vi "Data Server.vi"(8 "error in (no error)":errorcluster, 11 "Node Ptr":T1 format="%.0x") -> (0 "error out":errorcluster)   [LabVIEW 2021, in "gRPC Data Server System Explorer.lvlib"]
uses:
  gRPC Data Server System Explorer.lvlib
  <vilib>/NI VeriStand/Custom Device API/Custom Device Item Ref.ctl
  <vilib>/Utility/file.llb/Read Delimited Spreadsheet (string).vi
  <vilib>/Utility/file.llb/Write Delimited Spreadsheet (string).vi
  <vilib>/NI VeriStand/Custom Device API/Custom Device API.lvlib
  Shared/gRPC Data Server Shared.lvlib
panel:
  in  "Data":string[][](table)
  in  "Import":bool
  in  "Export":bool
  in  "SHDocVw.IWebBrowser":refnum<k7>(container)
  in  "Specific Header":cluster{"Section Name":string}={"Section Name"="Data in Memory"}
  in  "General Header":cluster{"Section Name":string}={"Section Name"="General Page Settings"}
  in  "Description":string
  in  "Name":string
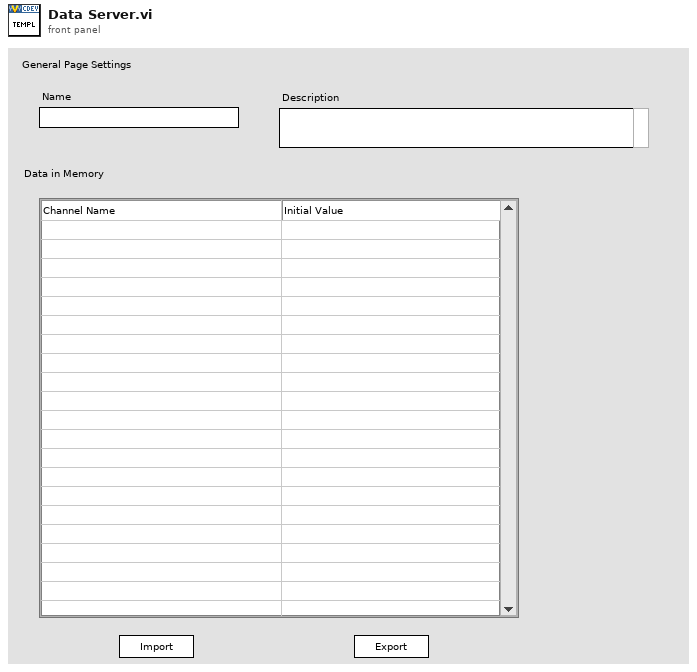
[diagram p1: front panel]
types:
  T1 = typedef "Custom Device API.lvlib/Custom Device Item Ref.ctl" = u64
  T2 = typedef "Custom Device API.lvlib/Custom Device Item Info.ctl" = cluster{"Name":string, "Is Channel":bool, "GUID":string, "Is Waveform":bool}
  T3 = typedef "gRPC Data Server Shared.lvlib/Compiled.Settings.ctl" = cluster{"Name":string, "Server Address":string, "Async?":bool, "Key File":path, "Cert File":path, "Channel Name":string[], "Initial Value":string[]}
  T4 = typedef "Custom Device API.lvlib/Custom Device Commands.ctl" = enum16{"Default", "Item renamed", "Shutdown", "Dynamic button pressed"}
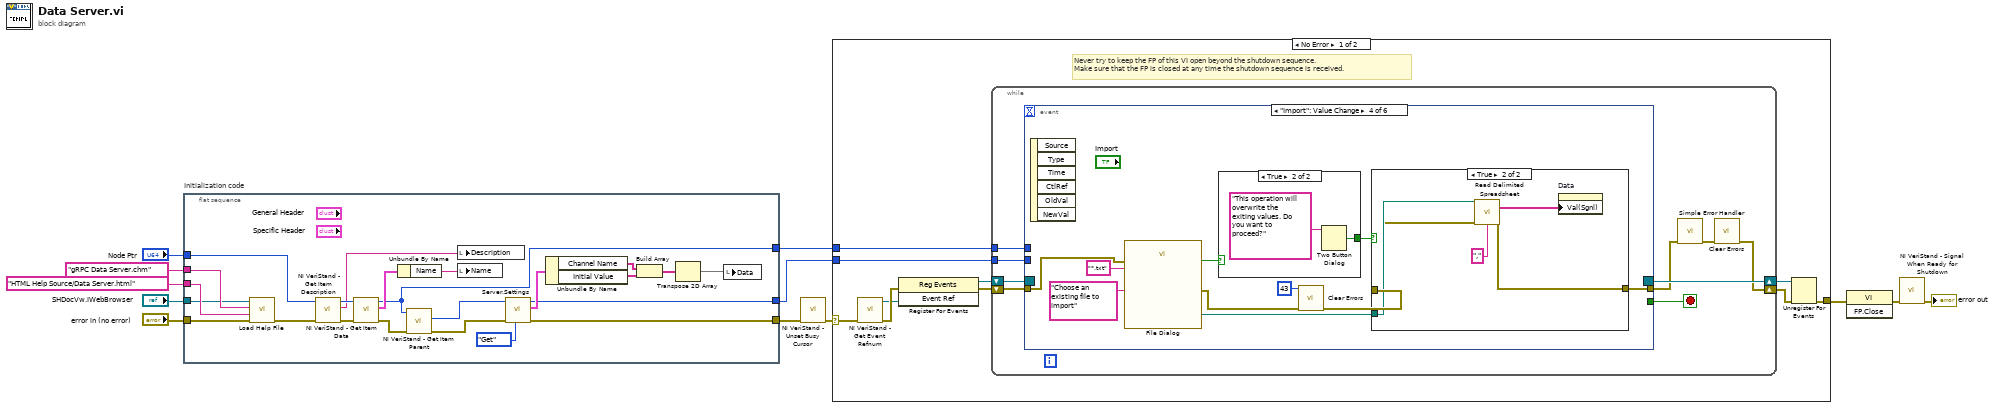
[diagram p0: block diagram]
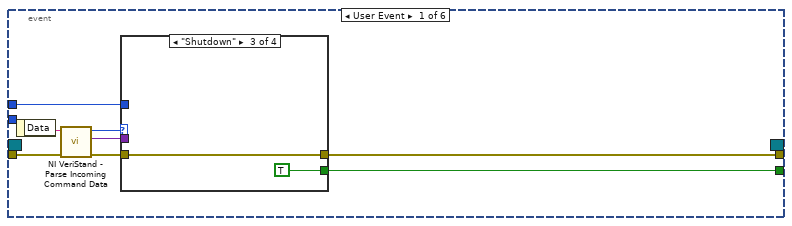
[diagram p2: hidden frame]
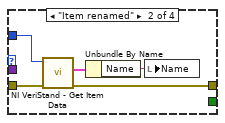
[diagram p4: hidden frame]
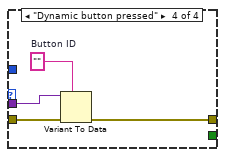
[diagram p5: hidden frame]
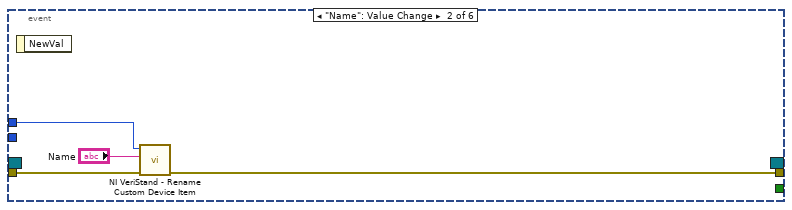
[diagram p6: hidden frame]
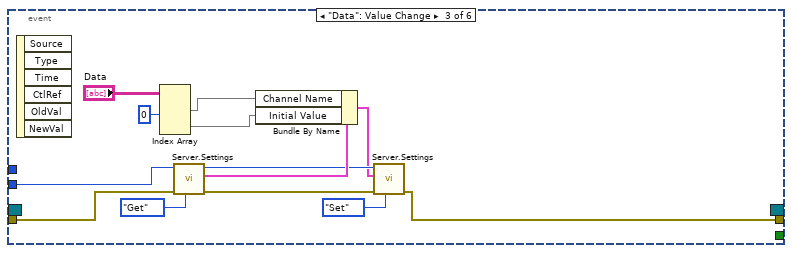
[diagram p7: hidden frame]
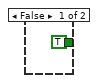
[diagram p9: hidden frame]
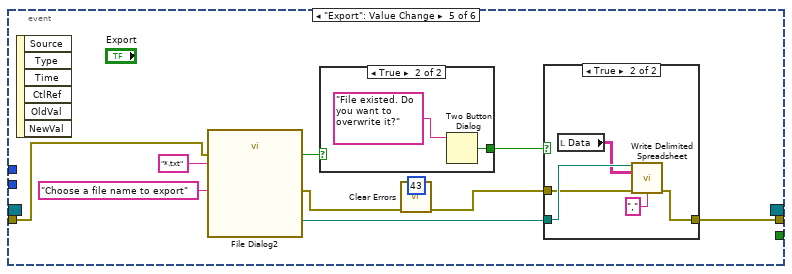
[diagram p10: hidden frame]
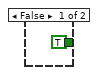
[diagram p12: hidden frame]
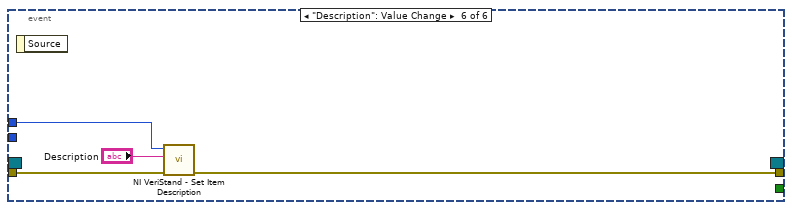
[diagram p13: hidden frame]
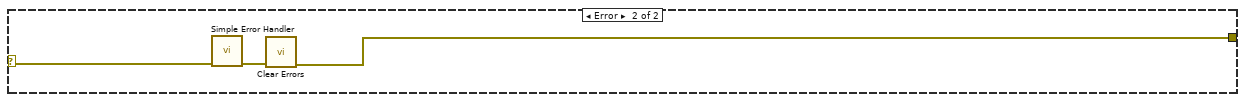
[diagram p14: hidden frame]
diagram:
  n1 = flat-sequence "Initialization code" {
    tunnel: "error in (no error)" -> [w29]
    tunnel: "Node Ptr" -> [w32]
    tunnel: [w23] -> w8
    tunnel: [w17] -> w5
    tunnel: "SHDocVw.IWebBrowser" -> [w25]
    tunnel: "HTML Help Source/Data Server.html" ("CD_CHM_Section") -> [w27]
    tunnel: "gRPC Data Server.chm" ("CD_CHM_FileName") -> [w26]
    tunnel: [w13] -> w1
    frame #0 {
      n2 = call "Load Help File.vi"("error in (no error)"=w29, "HTML File to Load"=w27, "Main CHM File"=w26, "Browser"=w25) -> ("error out"=w28:errorcluster)  [unwired: 7 in]
      n3 = call <vilib>:"NI VeriStand - Get Item Description.vi"("error in (no error)"=w28, "Item Ref in"=w32) -> ("error out"=w34:errorcluster, "Description"=w30:string, "Item Ref out"=w35:T1)  [unwired: 7 out]
      n4 = call <vilib>:"NI VeriStand - Get Item Data.vi"("error in (no error)"=w34, "Item Ref in"=w35) -> ("error out"=w16:errorcluster, "Item Info"=w33:T2, "Item Ref out"=w17:T1)  [unwired: 7 out]
      n5 = Unbundle By Name(w33) -> ("Name"=w31:string)
      n6 = call <vilib>:"NI VeriStand - Get Item Parent.vi"("error in (no error)"=w16, "Item Ref in"=w17) -> ("error out"=w14:errorcluster, "Parent Ref"=w15:T1)  [unwired: 6 in, 2 out]
      n7 = local write "Description"(w30) -> ()
      n8 = local write "Name"(w31) -> ()
      n9 = call "Server.Settings.vi"("Action"=enum8{"Get", "Set"}."Get", "error in (no error)"=w14, "Parent Ref in"=w15) -> ("error out"=w23:errorcluster, "Settings Out"=w22:T3, "Item Ref out"=w13:T1)  [unwired: 6 in]
      n10 = Unbundle By Name(w22) -> ("Channel Name"=w21:string[], "Initial Value"=w20:string[])
      n11 = Build Array(w21, w20) -> (w19:string[][])
      n12 = Transpose 2D Array(2D array=w19) -> (transposed array=w18:string[][])
      n13 = local write "Data"(w18) -> ()
    }
  }
  n14 = call <vilib>:"NI VeriStand - Unset Busy Cursor.vi"("error in (no error)"=w8) -> ("error out"=w7:errorcluster)  [unwired: 10 out]
  n15 = case shown="No Error" w7 {
    selector: w7 -> [w37 w136]
    tunnel: [w42 w134] -> w12
    tunnel: w5 -> [w38 _]
    tunnel: w1 -> [w36 _]
    frame No Error {
      # "Never try to keep the FP of this VI open beyond the shutdown sequence.\nMake sure that the FP is closed at any time the shutdown sequence is received."
      n16 = call <vilib>:"NI VeriStand - Get Event Refnum.vi"("error in (no error)"=w37) -> ("error out"=w45:errorcluster, "Event Ref"=w41:refnum<user-event>)  [unwired: 9 out]
      n17 = register-events(error in=w45, w41) -> (reference out=w39:refnum<event-registration>, error out=w40:errorcluster)  [unwired: 1 in]
      n18 = while {
        tunnel: w38 -> [w50]
        shift-right: [w47] -> w43
        shift-left: w40 -> [w53]
        shift-right: [w54] -> w44
        shift-left: w39 -> [w52]
        tunnel: w36 -> [w46]
        stop <- w51 stop-if-true
        n19 = event shown="[3] \"Import\": Value Change" {
          selector: w52 -> [_ _ _ _ _ _]
          dyn-events: [_ _ _ _ _ _] -> w54
          timeout: _ -> [_ _ _ _ _ _]
          tunnel: w53 -> [w62 w78 w85 w99 w115 w132]
          tunnel: [w58 _ _ _ _ _] -> w51
          tunnel: [w57 w77 w84 w95 w114 w131] -> w49
          tunnel: w50 -> [w56 w76 _ _ _ w133]
          tunnel: w46 -> [_ _ w79 _ _ _]
          event User Event {
            n20 = event-data() -> ("Data"=w61:string)  [unwired: 1 out]
            n21 = call <vilib>:"NI VeriStand - Parse Incoming Command Data.vi"("error in (no error)"=w62, "Incoming data"=w61) -> ("error out"=w60:errorcluster, "Outgoing data"=w55:variant, "Action"=w59:T4)  [unwired: 7 out]
            n22 = case shown="\"Shutdown\"" w59 {
              tunnel: w60 -> [w63 w68 w69 w74]
              tunnel: [_ _ TRUE _] -> w58
              tunnel: [w63 w65 w69 w71] -> w57
              tunnel: w56 -> [_ w67 _ _]
              tunnel: w55 -> [_ _ _ w73]
              frame "Default", Default {
              }
              frame "Item renamed" {
                n23 = call <vilib>:"NI VeriStand - Get Item Data.vi"("error in (no error)"=w68, "Item Ref in"=w67) -> ("error out"=w65:errorcluster, "Item Info"=w66:T2)  [unwired: 8 out]
                n24 = Unbundle By Name(w66) -> ("Name"=w64:string)
                n25 = local write "Name"(w64) -> ()
              }
              frame "Shutdown" {
              }
              frame "Dynamic button pressed" {
                w72 = ""  # Button ID
                n26 = Variant To Data(error in=w74, type=w72, Variant=w73) -> (error out=w71:errorcluster)  [unwired: 1 out]
              }
            }
          }
          event "Name": Value Change {
            n27 = event-data() -> ()  [unwired: 2 out]
            n28 = call <vilib>:"NI VeriStand - Rename Custom Device Item.vi"("error in (no error)"=w78, "New Name"="Name", "Item Ref in"=w76) -> ("error out"=w77:errorcluster)  [unwired: 1 in, 7 out]
          }
          event "Data": Value Change {
            n29 = event-data() -> ()  [unwired: 7 out]
            n30 = Index Array(array="Data", index (col) #1=0 ("disabled index (col)")) -> (element #1=w81:string[], element #2=w80:string[])  [unwired: 3 in]
            n31 = call "Server.Settings.vi"("Action"=enum8{"Get", "Set"}."Get", "error in (no error)"=w85, "Parent Ref in"=w79) -> ("error out"=w88:errorcluster, "Settings Out"=w90:T3, "Item Ref out"=w89:T1)  [unwired: 6 in]
            n32 = Bundle By Name(cluster=w90, "Channel Name"=w81, "Initial Value"=w80) -> (w87:T3)
            n33 = call "Server.Settings.vi"("Action"=enum8{"Get", "Set"}."Set", "error in (no error)"=w88, "Settings In"=w87, "Parent Ref in"=w89) -> ("error out"=w84:errorcluster)  [unwired: 5 in, 2 out]
          }
          event "Import": Value Change {
            n34 = event-data() -> ()  [unwired: 7 out]
            n35 = call "File Dialog"("prompt"="Choose an existing file to import", "error in"=w99, "pattern (all files)"="*.txt" ("default name")) -> ("selected path"=w96:path, "exists"=w97:bool, "error out"=w94:errorcluster)  [unwired: 9 in, 1 out]
            n36 = case shown="True" w97 {
              tunnel: [TRUE ("T button?") w109] -> w98
              frame False {
              }
              frame True {
                n37 = Two Button Dialog(message="This operation will overwrite the exiting values. Do you want to proceed?") -> (T button?=w109:bool)  [unwired: 2 in]
              }
            }
            n38 = call <vilib>:"Clear Errors.vi"("error in (no error)"=w94, "specific error code to clear (0: all)"=43) -> ("error out"=w93:errorcluster)  [unwired: 4 in, 1 out]
            n39 = case shown="True" w98 {
              tunnel: w96 -> [_ w107]
              tunnel: w93 -> [w102 w105]
              tunnel: [w102 w104] -> w95
              frame False {
              }
              frame True {
                n40 = call-poly <vilib>:"Read Delimited Spreadsheet.vi"("file path (dialog if empty)"=w107, "error in (no error)"=w105, "delimiter (\\t)"="," ("delimiter (\\t)")) -> ("all rows"=w103:string[][], "error out"=w104:errorcluster)  [unwired: 7 in, 4 out]
                n41 = property on="Data" class="Tbl (strict)"("Val(Sgnl)"=w103) -> ()  [unwired: 2 in, 2 out]
              }
            }
          }
          event "Export": Value Change {
            n42 = event-data() -> ()  [unwired: 7 out]
            n43 = call "File Dialog2"("prompt"="Choose a file name to export", "error in"=w115, "pattern (all files)"="*.txt" ("default name")) -> ("selected path"=w116:path, "exists"=w118:bool, "error out"=w112:errorcluster)  [unwired: 9 in, 1 out]
            n44 = case shown="True" w118 {
              tunnel: [TRUE ("T button?") w128] -> w117
              frame False {
              }
              frame True {
                n45 = Two Button Dialog(message="File existed. Do you want to overwrite it?") -> (T button?=w128:bool)  [unwired: 2 in]
              }
            }
            n46 = call <vilib>:"Clear Errors.vi"("error in (no error)"=w112, "specific error code to clear (0: all)"=43) -> ("error out"=w111:errorcluster)  [unwired: 4 in, 1 out]
            n47 = case shown="True" w117 {
              tunnel: w116 -> [_ w126]
              tunnel: w111 -> [w121 w123]
              tunnel: [w121 w122] -> w114
              frame False {
              }
              frame True {
                n48 = local read "Data"() -> (w124:string[][])
                n49 = call-poly <vilib>:"Write Delimited Spreadsheet.vi"("file path (dialog if empty)"=w126, "2D data"=w124, "error in (no error)"=w123, "delimiter (\\t)"="," ("delimiter (\\t)")) -> ("error out"=w122:errorcluster)  [unwired: 10 in, 1 out]
              }
            }
          }
          event "Description": Value Change {
            n50 = event-data() -> ()  [unwired: 2 out]
            n51 = call <vilib>:"NI VeriStand - Set Item Description.vi"("error in (no error)"=w132, "Description"="Description", "Item Ref in"=w133) -> ("error out"=w131:errorcluster)  [unwired: 8 out]
          }
        }
        n52 = call <vilib>:"Simple Error Handler.vi"("error in (no error)"=w49) -> ("error out"=w48:errorcluster)  [unwired: 1 in, 7 out]
        n53 = call <vilib>:"Clear Errors.vi"("error in (no error)"=w48) -> ("error out"=w47:errorcluster)  [unwired: 1 in, 5 out]
      }
      n54 = Unregister For Events(event registration refnum=w44, error in=w43) -> (error out=w42:errorcluster)
    }
    frame Error {
      n55 = call <vilib>:"Simple Error Handler.vi"("error in (no error)"=w136) -> ("error out"=w135:errorcluster)  [unwired: 1 in, 7 out]
      n56 = call <vilib>:"Clear Errors.vi"("error in (no error)"=w135) -> ("error out"=w134:errorcluster)  [unwired: 1 in, 5 out]
    }
  }
  n57 = invoke class="VI" method="FP.Close"(error in=w12) -> (error out=w11:errorcluster)  [unwired: 2 in, 2 out]
  n58 = call <vilib>:"NI VeriStand - Signal When Ready for Shutdown.vi"("error in (no error)"=w11) -> ("error out"=→"error out":errorcluster)  [unwired: 10 out]
